vi "SampleGetIDMultiple.vi"() -> ()   [LabVIEW 2013]
uses:
  C:/Users/Saffmanlab/Documents/git/CsPyController/labview/cesium_controller/PicoMotor/NewFocus8742/CmdLib.dll
  CmdLib.dll
panel:
  out "Identification List":string[](array[string])
  out "DeviceKey List Out":string[](array[string])
  out "error out":errorcluster
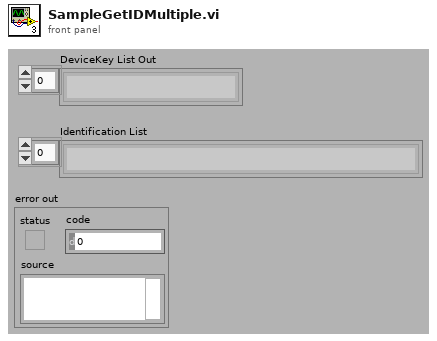
[diagram p1: front panel]
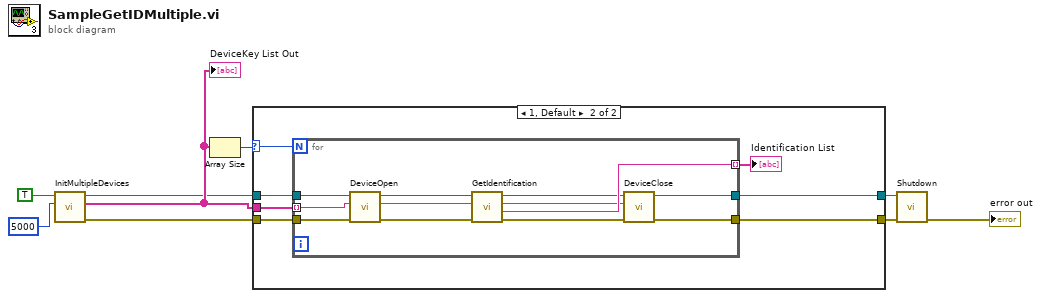
[diagram p0: block diagram]
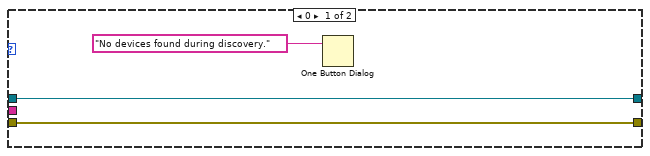
[diagram p2: hidden frame]
diagram:
  n1 = call "InitMultipleDevices.vi"("msecDelayForDiscovery"=5000, "logging"=TRUE) -> ("error out"=w3:errorcluster, "DeviceKey List Out"=w5:string[], "CmdLib Out"=w4:refnum<k24>)  [unwired: 3 in]
  "DeviceKey List Out" <- w5
  n2 = Array Size(array=w5) -> (size(s)=w6:i32)
  n3 = case shown="1, Default" w6 {
    selector: w6 -> [_ w19]
    tunnel: w5 -> [_ w18]
    tunnel: w4 -> [w11 w17]
    tunnel: w3 -> [w12 w16]
    tunnel: [w12 w15] -> w2
    tunnel: [w11 w14] -> w1
    frame 0 {
      n4 = One Button Dialog(message="No devices found during discovery.") -> ()  [unwired: 1 in, 1 out]
    }
    frame 1, Default {
      n5 = for {
        N: w19 -> [_]
        tunnel: w18 -> [w26] mode=indexing
        tunnel: [w31] -> w13 mode=indexing
        tunnel: w17 -> [w30]
        tunnel: w16 -> [w24]
        tunnel: [w22] -> w15
        tunnel: [w28] -> w14
        n6 = call "DeviceOpen.vi"("error in (no error)"=w24, "DeviceKey In"=w26, "CmdLib In"=w30) -> ("error out"=w23:errorcluster, "DeviceKey Out"=w25:string, "CmdLib Out"=w29:refnum<k24>)  [unwired: 2 in]
        n7 = call "GetIdentification.vi"("error in (no error)"=w23, "DeviceKey In"=w25, "CmdLib In"=w29) -> ("error out"=w21:errorcluster, "Identification"=w31:string, "DeviceKey Out"=w20:string, "CmdLib Out"=w27:refnum<k24>)  [unwired: 1 in]
        n8 = call "DeviceClose.vi"("error in (no error)"=w21, "DeviceKey In"=w20, "CmdLib In"=w27) -> ("error out"=w22:errorcluster, "CmdLib Out"=w28:refnum<k24>)  [unwired: 2 in, 1 out]
      }
      "Identification List" <- w13
    }
  }
  n9 = call "Shutdown.vi"("error in (no error)"=w2, "CmdLib In"=w1) -> ("error out"=→"error out":errorcluster)  [unwired: 4 in, 1 out]
